vi "Process_DAQ.vi"(8 "error in (no error)":errorcluster, 9 "start process sync notifier":refnum<notifier>, 10 "TopLevel":refnum<class "TopLevel.lvclass">, 11 "DAQ":refnum<class "DAQ.lvclass">) -> (0 "error out":errorcluster)   [LabVIEW 2022 SP3, in "DAQ.lvclass"]
doc: "Developed by Kevin Thompson\nkevin@thompsonengineering.net\n\nCopyright 2015\nThompson Engineering, LLC"
uses:
  DAQ.lvclass
  TopLevel/TopLevel.lvclass
  Process_DAQ SM AppData--cluster.ctl
  DataTypes/TD DAQ Settings--cluster.ctl
  DataTypes/TD DI Instrument Settings--cluster.ctl
  DataTypes/TD AI Instrument Settings--cluster.ctl
  DataTypes/TD AI InstSettings--cluster.ctl
  ProcessSupport/TD SimAI Ranges--cluster.ctl
  <vilib>/TELLC/Dynamic CVT API/TD Dynamic CVT DVR--ref.ctl
  DAQ.lvclass/DAQ.ctl
  ProcessSupport/TD DAQ Output Cmd EventData--cluster.ctl
  ProcessSupport/TD DaqOutCmd--enum.ctl
  DataTypes/TD DAQ Output EventSenderMode-enum.ctl
  DataTypes/TD DO Channel--cluster.ctl
  DataTypes/TD AO Channel--cluster.ctl
  DataTypes/TD DataValueConversion--cluster.ctl
  DataTypes/AsyncCmd_DAQ--enum.ctl
  Accessors/Get AI TaskNames.vi
  Accessors/Get DI TaskNames.vi
  Accessors/Get DAQ Settings.vi
  <vilib>/DAQmx/read.llb/DAQmx Read (Digital Bool 1Line 1Point).vi
  Accessors/Get IO Nodes.vi
  ProcessSupport/Get AI DAQ SMQ - array.vi
  ProcessSupport/Get DI DAQ SMQ - array.vi
  ProcessSupport/Get AI DAQ SMQ - single.vi
  <vilib>/DAQmx/miscellaneous.llb/DAQmx Fill In Error Info.vi
  DAQ_Common/Lib/ErrorHandler/ErrorHandler.lvclass
panel:
  in  "injected error cluster":errorcluster
  in  "inject error":bool
  out "time per buffer":dbl
  in  "Stop Process":bool
  # "Simulated error injection\nfor testing and debug"
  # "Makes sure to set this value from the process caller. Using the Start asyncronous call function."
  # "This is for debugging. Process should stop from user event."
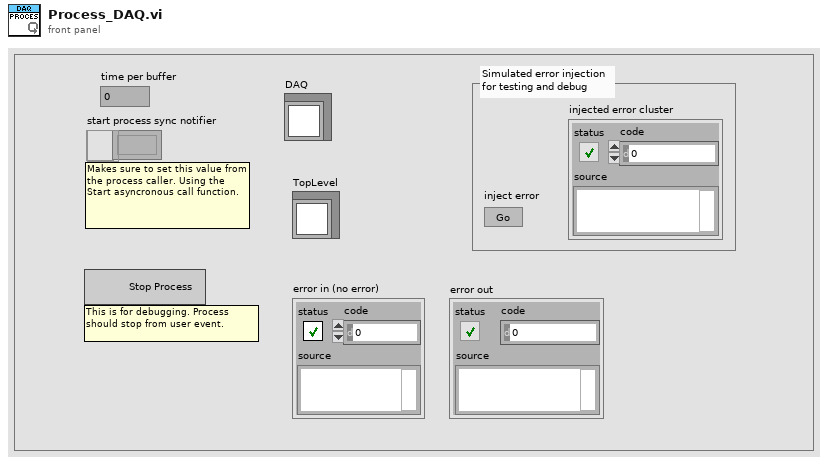
[diagram p1: front panel]
types:
  T1 = typedef "DAQ.lvclass/Process_DAQ SM AppData--cluster.ctl" = cluster{"Core":cluster{"Current VI Ref":refnum<vi>, "process sync notifier":refnum<notifier>}, "AsyncSMQ":refnum<queue>, "DAQ Settings":T2, "SimDaqLoopIntv":i32, "ThreadSyncRndzv":T7, "DAQ Node Dict DVR":T8, "DAQ Data Dict DVR":T8, "vData":variant, "quitting":bool, "Self Reference":refnum<class "DAQ.lvclass">, "AI Thread SMQs":variant, "AI TaskNames*":string[], "AI DAQ SMQ []":refnum<queue>[], "DI Thread SMQs":variant, "DI TaskNames*":string[], "DI DAQ SMQ []":refnum<queue>[]}
  T2 = typedef "DAQ.lvclass/TD DAQ Settings--cluster.ctl" = cluster{"Simulate DAQ":bool, "DI Settings":T3[], "AI Settings":T4[], "Relay IONames":string[], "AO IONames":string[], "AO NChan SingleTask":bool}
  T3 = typedef "DAQ.lvclass/TD DI Instrument Settings--cluster.ctl" = cluster{"Disable":bool, "DI TaskName":string, "DI RefreshIntv":i32}
  T4 = typedef "DAQ.lvclass/TD AI Instrument Settings--cluster.ctl" = cluster{"Disable":bool, "AI TaskName":string, "AI InstSettings":T5, "SimAI Ranges":T6}
  T5 = typedef "DAQ.lvclass/TD AI InstSettings--cluster.ctl" = cluster{"DaqRate":dbl, "NumSamples":i32}
  T6 = typedef "DAQ.lvclass/TD SimAI Ranges--cluster.ctl" = cluster{"lo":dbl, "hi":dbl}
  T7 = typedef "Rendezvous RefNum" = refnum<k1>
  T8 = typedef "TD Dynamic CVT DVR--ref.ctl" = refnum<data-value>
  T9 = typedef "DAQ.lvclass/TD DO Channel--cluster.ctl" = cluster{"DevName":string, "IOName":string, "IOPath":string, "SchemName":string, "logic":enum16{"Lo", "Hi"}, "DAQmx Task":refnum<k21>}
  T10 = typedef "DAQ.lvclass/TD DAQ Output Cmd EventData--cluster.ctl" = cluster{"TimeStamp":dbl, "DaqOutCmd":T11, "IOName":string, "BoolState":bool, "AnalogVal":dbl, "WaitTime (ms)":u32, "mode":T12, "vData":variant}
  T11 = typedef "DAQ.lvclass/TD DaqOutCmd--enum.ctl" = enum16{"Set DO", "Set AO", "Toggle DO", "Invert DO"}
  T12 = typedef "DAQ.lvclass/TD DAQ Output EventSenderMode-enum.ctl" = enum16{"manual", "automation"}
  T13 = typedef "DAQ.lvclass/TD AO Channel--cluster.ctl" = cluster{"DevName":string, "IOName":string, "IOPath":string, "SchemName":string, "Vmin":dbl, "Vmax":dbl, "Conversion":T14, "DAQmx Task":refnum<k21>}
  T14 = typedef "DAQ.lvclass/TD DataValueConversion--cluster.ctl" = cluster{"MaxSignal":dbl, "MinSignal":dbl, "MaxEngUnit":dbl, "MinEngUnit":dbl, "ScaleOffset":dbl, "negate":bool}
  T15 = typedef "DAQ.lvclass/AsyncCmd_DAQ--enum.ctl" = enum16{"StartDAQ", "StopDAQ", "CfgDAQ"}
  T16 = typedef "DAQ.lvclass/TD IO Node Definition--cluster.ctl" = cluster{"DI Config":T17, "DO Config":T20, "AI Config":T21, "AO Config":T26}
  T17 = typedef "DAQ.lvclass/TD DI Config--cluster.ctl" = cluster{"DI Tasks":T18[]}
  T18 = typedef "DAQ.lvclass/TD DI Task--cluster.ctl" = cluster{"DI TaskName":string, "DI Channels":T19[]}
  T19 = typedef "DAQ.lvclass/TD DI Channel--cluster.ctl" = cluster{"DevName":string, "IOName":string, "IOPath":string, "SchemName":string, "logic":enum16{"Lo", "Hi"}, "Index":i32}
  T20 = typedef "DAQ.lvclass/TD DO Config--cluster.ctl" = cluster{"DO Channels":T9[]}
  T21 = typedef "DAQ.lvclass/TD AI Config--cluster.ctl" = cluster{"AI Tasks":T22[]}
  T22 = typedef "DAQ.lvclass/TD AI Task--cluster.ctl" = cluster{"AI TaskName":string, "AI Channels":T23[]}
  T23 = typedef "DAQ.lvclass/TD AI Channel--cluster.ctl" = cluster{"DevName":string, "IOName":string, "IOPath":string, "SchemName":string, "MinValue":dbl, "MaxValue":dbl, "Terminal Configuration":i32, "Index":i32, "Conversion":T14, "AIType":T24, "Force Bridge":T25}
  T24 = typedef "DAQ.lvclass/TD AI DAQ Type--enum.ctl" = enum16{"Voltage", "Current", "Strain Gage", "Force Bridge"}
  T25 = typedef "DAQ.lvclass/TD AI Force Bridge--cluster.ctl" = cluster{"bridge information":cluster{"bridge configuration":i32, "voltage excitation source":i32, "voltage excitation value":dbl, "nominal bridge resistance":dbl}, "scaling information":cluster{"first electrical value":dbl, "second electrical value":dbl, "electrical units":i32, "first physical value":dbl, "second physical value":dbl, "physical units":i32}}
  T26 = typedef "DAQ.lvclass/TD AO Config--cluster.ctl" = cluster{"AO Channels":T13[]}
  T27 = typedef "TopLevel.lvclass/UserEvents.ctl" = cluster{"API Incoming Event":refnum<user-event>, "API Executed Event":refnum<user-event>, "API Return Event":refnum<user-event>, "Exit Event":refnum<user-event>, "StatusChanged":refnum<user-event>, "DLP GUI Config Changed":refnum<user-event>, "AppEvent":refnum<user-event>, "Login Event":refnum<user-event>, "HeadPrimeStatusEvent":refnum<user-event>}
  T28 = typedef "DAQ.lvclass/TD PublicEvents--cluster.ctl" = cluster{"DaqOutputCmd Ev":refnum<user-event>, "stop process":refnum<user-event>, "DAQ.AsyncCmd Event":refnum<user-event>, "DAQStateChanged Event":refnum<user-event>, "DAQ.AsyncMsg Event":refnum<user-event>, "DAQ_DO_StatusEvent":refnum<user-event>, "DIStateChangeEv":refnum<user-event>, "UI StateChanged":refnum<user-event>, "PurgeTimerEvent":refnum<user-event>}
  T29 = cluster{"AI InstSettings":T5, "AI TaskName":string}
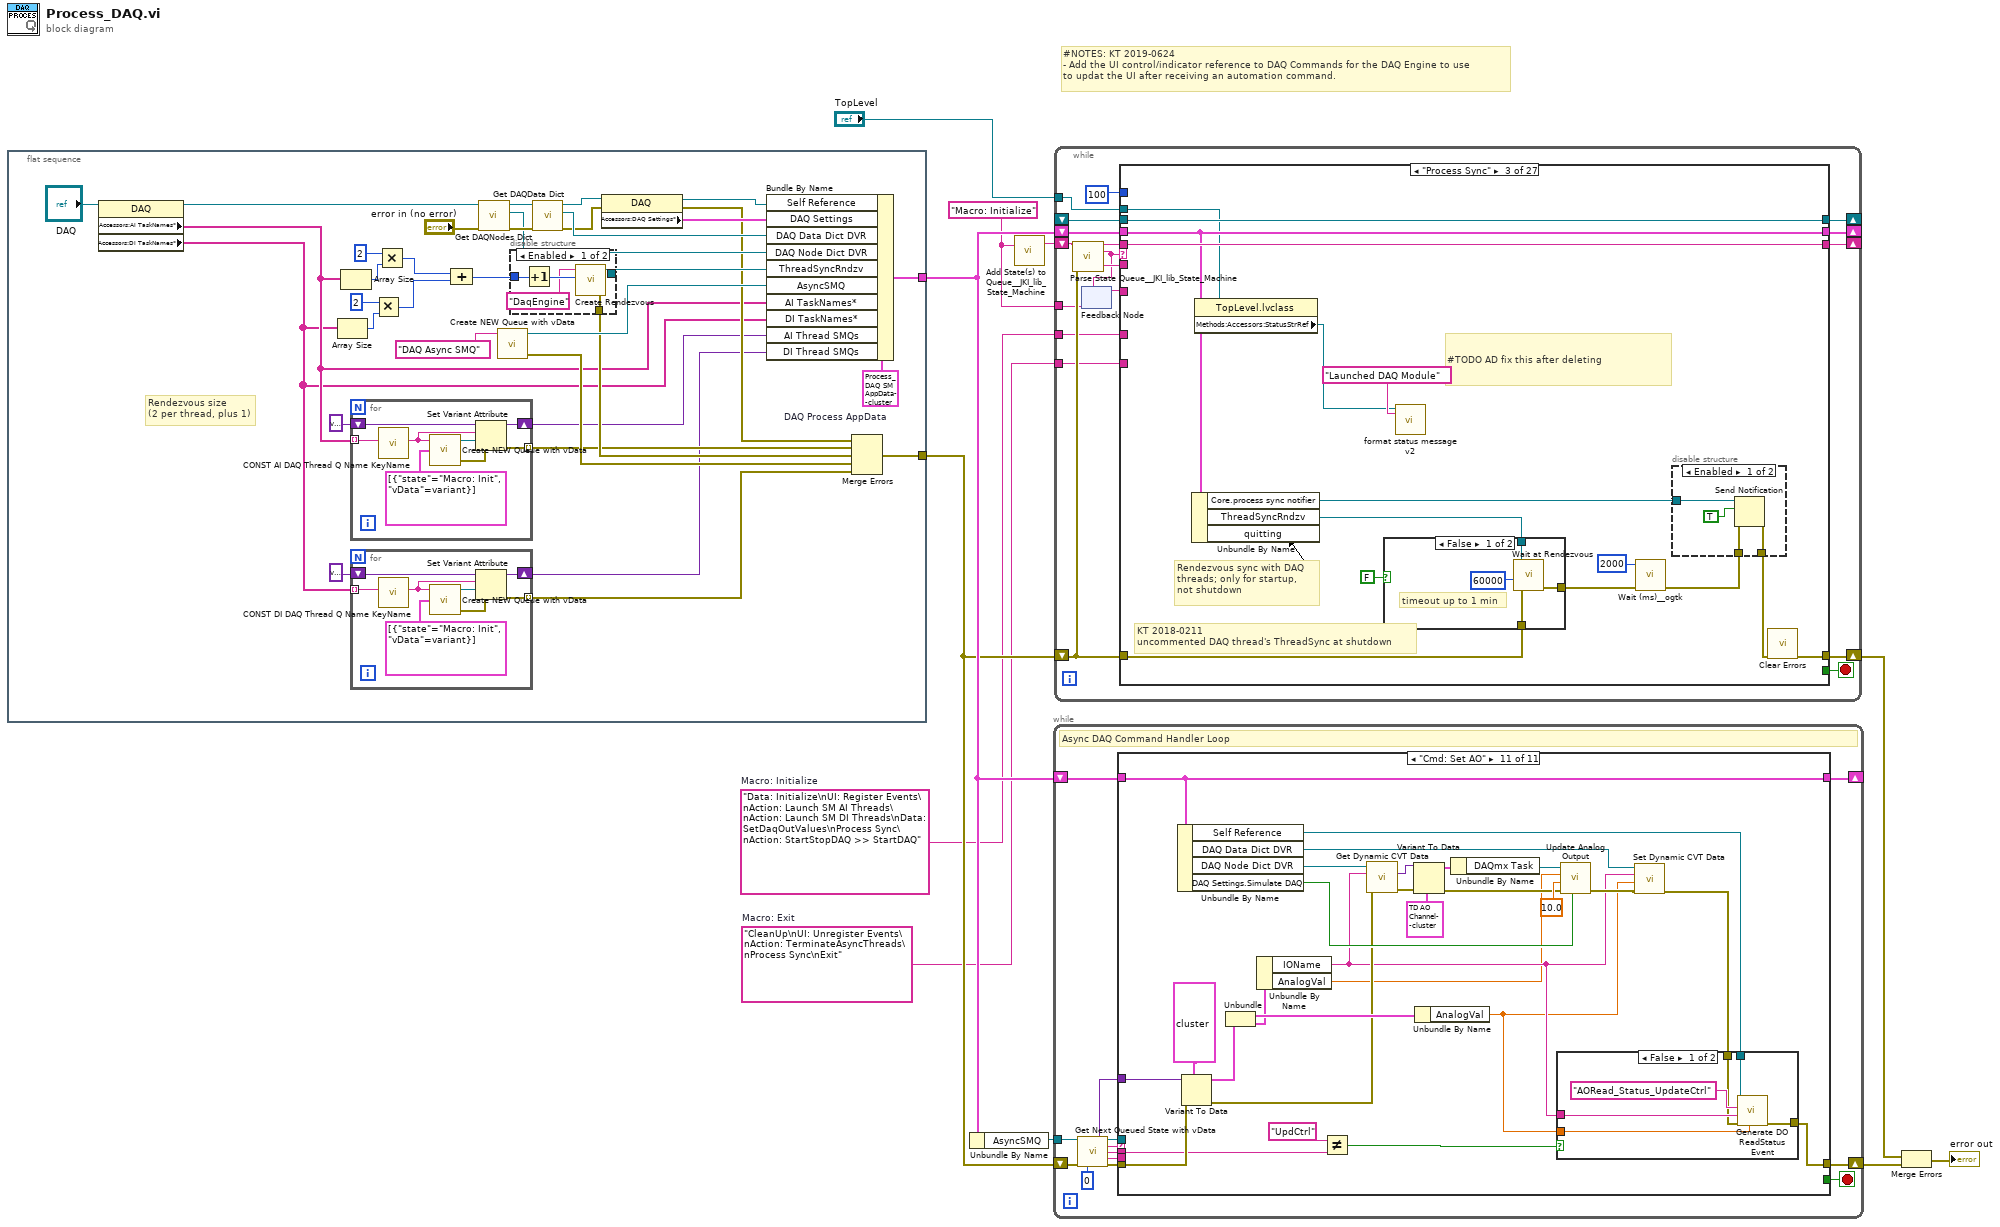
[diagram p0: block diagram]
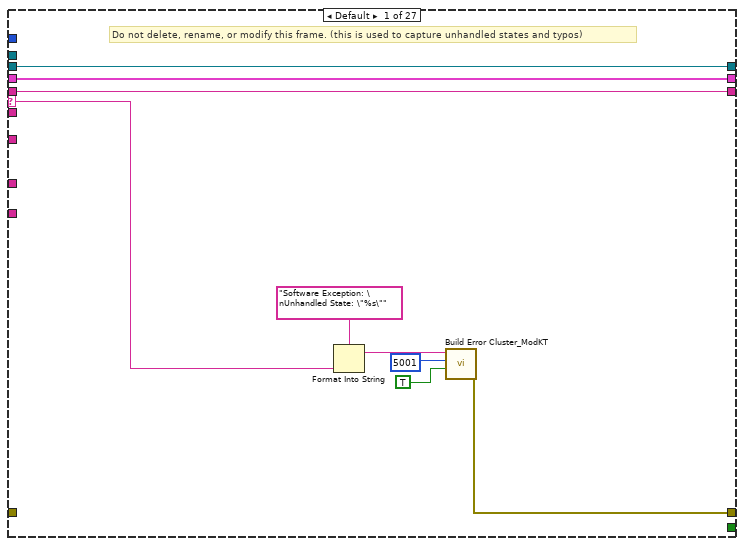
[diagram p2: hidden frame]
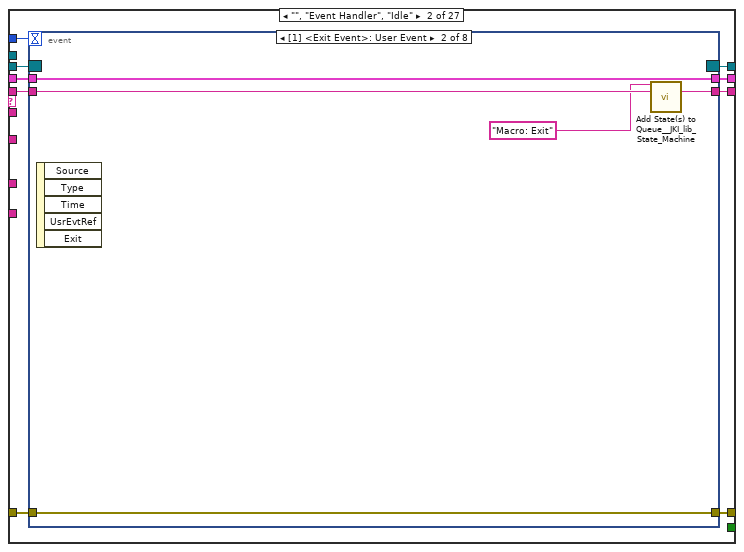
[diagram p3: hidden frame]
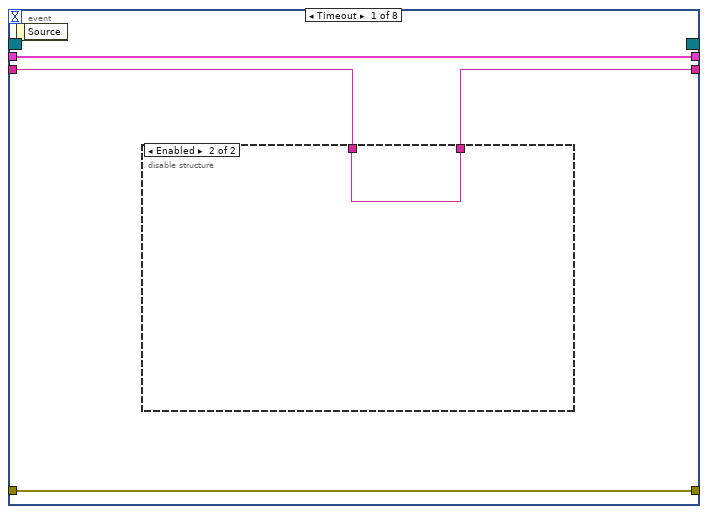
[diagram p4: hidden frame]
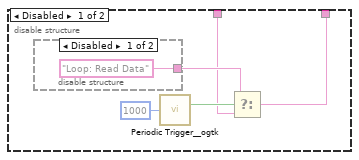
[diagram p5: hidden frame]
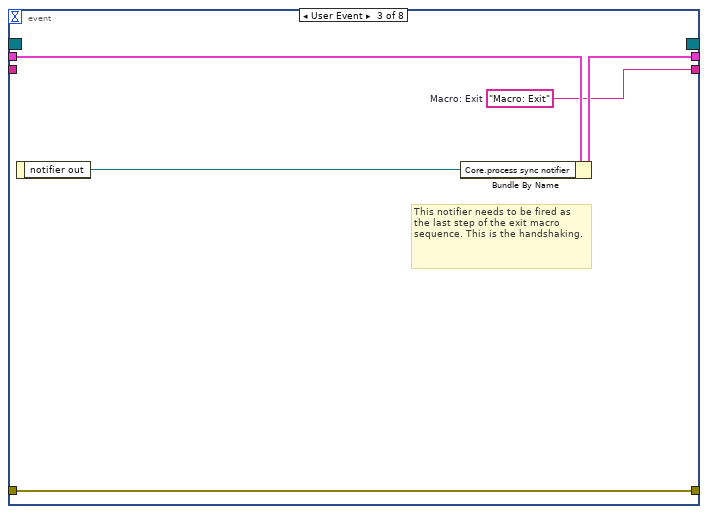
[diagram p7: hidden frame]
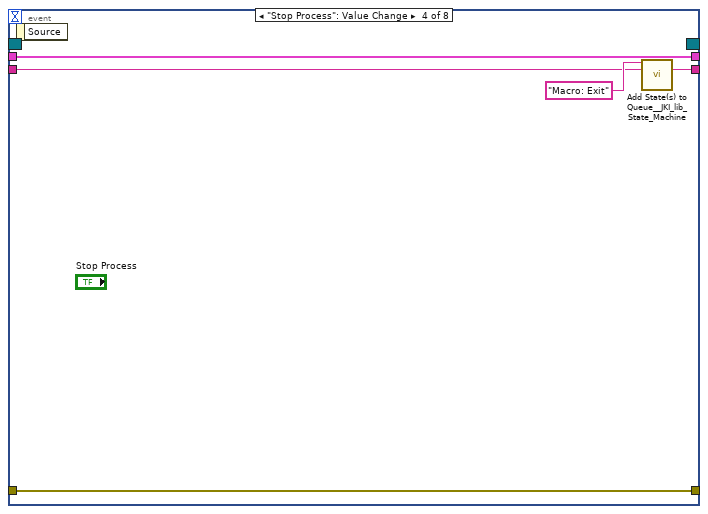
[diagram p8: hidden frame]
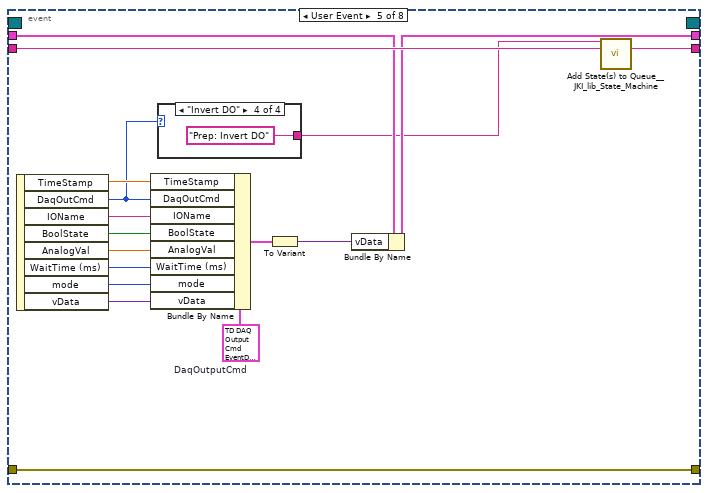
[diagram p9: hidden frame]
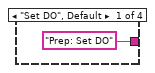
[diagram p10: hidden frame]
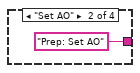
[diagram p11: hidden frame]
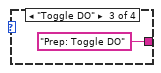
[diagram p12: hidden frame]
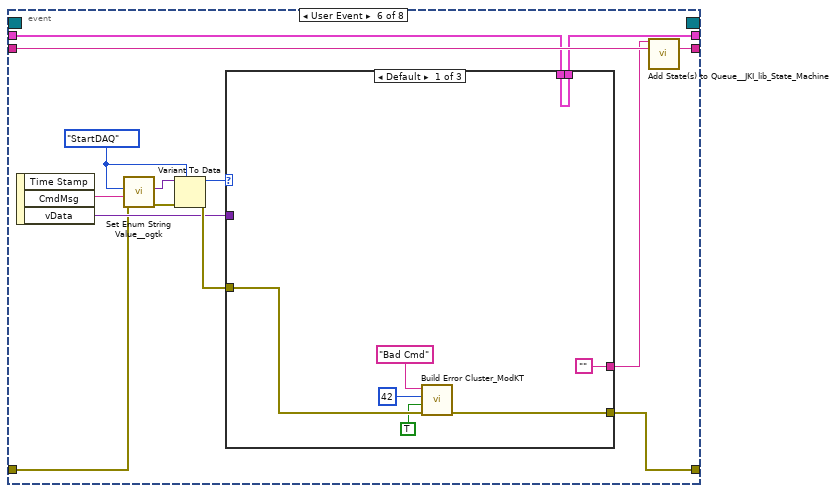
[diagram p13: hidden frame]
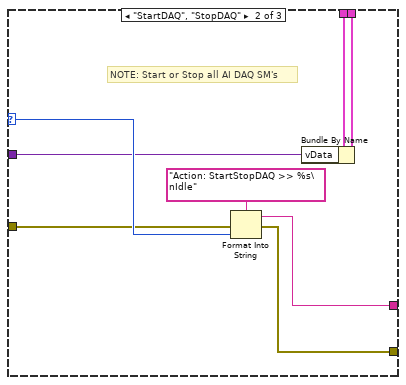
[diagram p14: hidden frame]
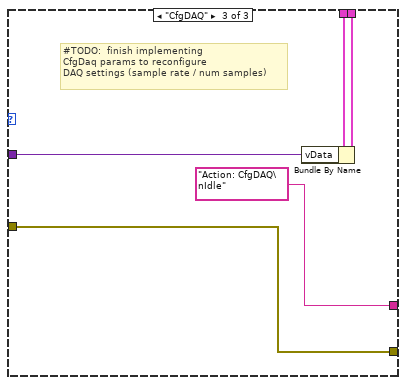
[diagram p15: hidden frame]
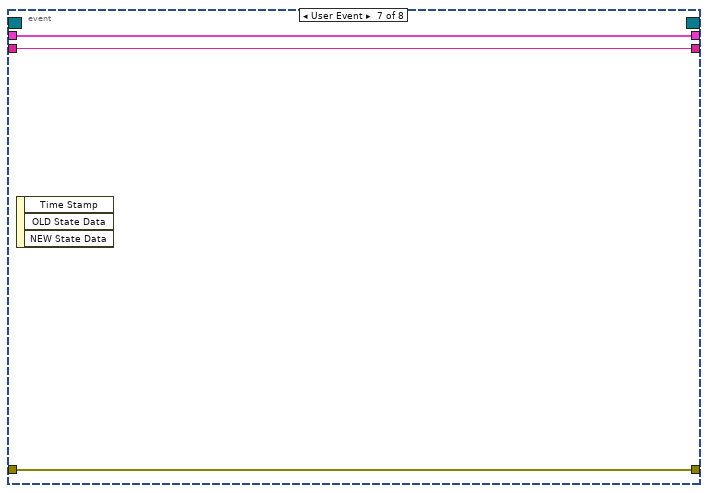
[diagram p16: hidden frame]
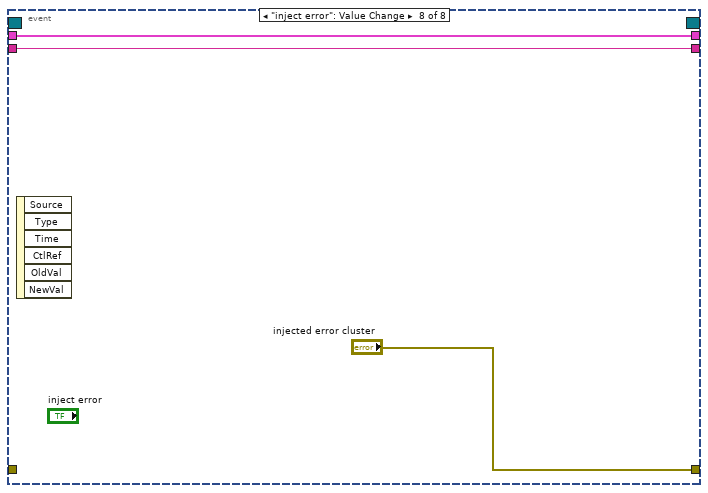
[diagram p17: hidden frame]
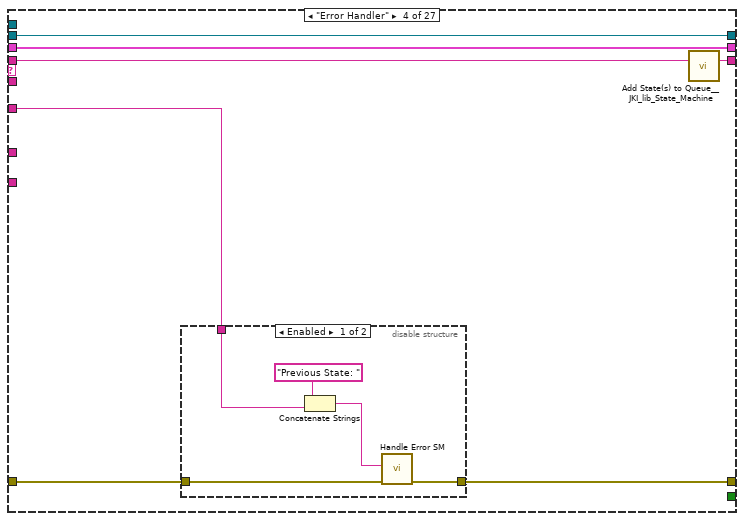
[diagram p20: hidden frame]
diagram:
  w4 = "Data: Initialize\nUI: Register Events\nAction: Launch SM AI Threads\nAction: Launch SM DI Threads\nData: SetDaqOutValues\nProcess Sync\nAction: StartStopDAQ >> StartDAQ"  # Macro: Initialize
  w3 = "CleanUp\nUI: Unregister Events\nAction: TerminateAsyncThreads\nProcess Sync\nExit"  # Macro: Exit
  w2 = "Macro: Initialize"
  # "#NOTES: KT 2019-0624\n- Add the UI control/indicator reference to DAQ Commands for the DAQ Engine to use\nto updat the UI after receiving an automation command."
  n1 = flat-sequence {
    tunnel: [w45] -> w9
    tunnel: [w35] -> w8
    frame #0 {
      w46 = T1 {"Core"={"Current VI Ref"=refnum, "process sync notifier"=refnum}, "AsyncSMQ"=refnum, "DAQ Settings"={"Simulate DAQ"=FALSE, "DI Settings"=[], "AI Settings"=[], "Relay IONames"=[], "AO IONames"=[], "AO NChan SingleTask"=FALSE}, "SimDaqLoopIntv"=0, "ThreadSyncRndzv"=refnum, "DAQ Node Dict DVR"=refnum, "DAQ Data Dict DVR"=refnum, "vData"=variant, "quitting"=FALSE, "Self Reference"=refnum, "AI Thread SMQs"=variant, "AI TaskNames*"=[], "AI DAQ SMQ []"=[], "DI Thread SMQs"=variant, "DI TaskNames*"=[], "DI DAQ SMQ []"=[]}  # DAQ Process AppData
      # "Rendezvous size\n(2 per thread, plus 1)"
      n2 = property class="DAQ"(reference="DAQ") -> (reference out=w26:refnum<class "DAQ.lvclass">, "Accessors:AI TaskNames*"=w23:string[], "Accessors:DI TaskNames*"=w13:string[])  [unwired: 1 in, 1 out]
      n3 = Array Size(array=w13) -> (size(s)=w18:i32)
      n4 = Array Size(array=w23) -> (size(s)=w22:i32)
      n5 = for {
        tunnel: [w65] -> w32 mode=indexing
        shift-right: [w64] -> w24
        shift-left: variant -> [w66]
        tunnel: w23 -> [w61] mode=indexing
        n6 = call "CONST AI DAQ Thread Q Name KeyName.vi"("AI TaskName"=w61) -> ("AI SMQ (KeyName)"=w63:string)  [unwired: 10 in]
        n7 = call <vilib>:"Create NEW Queue with vData.vi"("Initial States"=cluster{"state":string, "vData":variant}[] [{"state"="Macro: Init", "vData"=variant}], "Name (SMQ)"=w63) -> ("error out"=w60:errorcluster, "queue out"=w67:refnum<queue>)  [unwired: 2 in]
        n8 = Set Variant Attribute(Variant=w66, name=w63, value=w67, error in=w60) -> (Variant out=w64:variant, error out=w65:errorcluster)  [unwired: 1 out]
      }
      n9 = for {
        tunnel: [w57] -> w14 mode=indexing
        shift-right: [w56] -> w12
        shift-left: variant -> [w58]
        tunnel: w13 -> [w53] mode=indexing
        n10 = call "CONST DI DAQ Thread Q Name KeyName.vi"("DI TaskName"=w53) -> ("DI SMQ (KeyName)"=w55:string)  [unwired: 10 in]
        n11 = call <vilib>:"Create NEW Queue with vData.vi"("Initial States"=cluster{"state":string, "vData":variant}[] [{"state"="Macro: Init", "vData"=variant}], "Name (SMQ)"=w55) -> ("error out"=w52:errorcluster, "queue out"=w59:refnum<queue>)  [unwired: 2 in]
        n12 = Set Variant Attribute(Variant=w58, name=w55, value=w59, error in=w52) -> (Variant out=w56:variant, error out=w57:errorcluster)  [unwired: 1 out]
      }
      n13 = Multiply(x=2, y=w18) -> (x*y=w16:i32)
      n14 = Multiply(x=2, y=w22) -> (x*y=w20:i32)
      n15 = Compound Arithmetic op=ADD(w20, w16) -> (w17:i32)
      n16 = call "Get DAQNodes Dict.vi"("error in (no error)"="error in (no error)", "DAQ"=w26) -> ("error out"=w39:errorcluster, "DAQ Node Dict DVR"=w38:T8, "DAQ"=w41:refnum<class "DAQ.lvclass">)  [unwired: 7 in]
      n17 = call <vilib>:"Create NEW Queue with vData.vi"("Name (SMQ)"="DAQ Async SMQ") -> ("error out"=w43:errorcluster, "queue out"=w42:refnum<queue>)  [unwired: 3 in]
      n18 = disable-structure shown="Enabled" {
        disable-tunnel: [w51 _] -> w37
        disable-tunnel: [w50 _] -> w36
        disable-tunnel: w17 -> [w47 _]
        frame Enabled {
          n19 = Increment(x=w47) -> (x+1=w49:i32)
          n20 = call <vilib>:"Create Rendezvous.vi"("size (2)"=w49, "name (unnamed)"="DaqEngine" ("ProcVI ID")) -> ("error out"=w50:errorcluster, "rendezvous"=w51:T7)  [unwired: 3 in, 1 out]
        }
        frame Disabled {
        }
      }
      n21 = call "Get DAQData Dict.vi"("error in (no error)"=w39, "DAQ"=w41) -> ("error out"=w28:errorcluster, "DAQ Data Dict DVR"=w40:T8, "DAQ"=w31:refnum<class "DAQ.lvclass">)  [unwired: 7 in]
      n22 = property class="DAQ"(reference=w31, error in=w28) -> (reference out=w29:refnum<class "DAQ.lvclass">, error out=w25:errorcluster, "Accessors:DAQ Settings*"=w30:T2)
      n23 = Bundle By Name(cluster=w46, "Self Reference"=w29, "DAQ Settings"=w30, "DAQ Data Dict DVR"=w40, "DAQ Node Dict DVR"=w38, "ThreadSyncRndzv"=w37, "AsyncSMQ"=w42, "AI TaskNames*"=w23, "DI TaskNames*"=w13, "AI Thread SMQs"=w24, "DI Thread SMQs"=w12) -> (w45:T1)
      n24 = Merge Errors(w25, w32, w36, w43, w14) -> (w35:errorcluster)
    }
  }
  n25 = Unbundle By Name(w9) -> ("AsyncSMQ"=w10:refnum<queue>)
  n26 = call <vilib>:"Add State(s) to Queue__JKI_lib_State_Machine.vi"("State(s) in (\"\")"=w2) -> ("States Out"=w11:string)  [unwired: 14 in]
  n27 = while {
    shift-right: [w69] -> _
    shift-left: w9 -> [w70]
    tunnel: w10 -> [w80]
    shift-right: [w72] -> w7
    shift-left: w8 -> [w74]
    stop <- w71 stop-if-true
    # "Async DAQ Command Handler Loop"
    n28 = call <vilib>:"Get Next Queued State with vData.vi"("queue in"=w80, "error in (no error)"=w74, "timeout (100)"=0) -> ("vData out"=w75:variant, "queue out"=w78:refnum<queue>, "Next State"=w79:string, "queued msg"=w77:string, "Prev State"=w76:string, "error out"=w73:errorcluster)  [unwired: 6 in, 1 out]
    n29 = case shown="\"Cmd: Set AO\"" w79 {
      tunnel: w73 -> [_ w90 w100 _ w108 w115 w118 w138 w182 w228 w272]
      tunnel: w78 -> [_ _ _ w104 w109 _ _ _ _ _ _]
      tunnel: w77 -> [_ _ _ _ _ _ _ w134 w178 w224 w252]
      selector: w79 -> [w81 _ _ _ _ _ _ _ _ _ _]
      tunnel: w76 -> [_ w89 _ _ _ _ _ _ _ _ _]
      tunnel: w75 -> [_ _ _ _ _ _ _ w139 w183 w229 w271]
      tunnel: [w82 w88 w100 w106 w108 w114 w118 w122 w171 w215 w247] -> w72
      tunnel: [_ _ _ _ TRUE _ _ _ _ _ _] -> w71
      tunnel: w70 -> [w87 w91 w99 w107 w111 w116 w117 w137 w181 w227 w255]
      tunnel: [w87 w91 w99 w107 w111 w116 w117 w137 w181 w227 w255] -> w69
      frame Default {
        n30 = Format Into String(format string="Software Exception: \nUnhandled State: \"%s\"", w81) -> (resulting string=w84:string)  [unwired: 2 in, 1 out]
        n31 = call <vilib>:"Build Error Cluster_ModKT .vi"("Prepend String (\"\")"=w84, "code"=5001, "error? (F)"=TRUE ("error?")) -> ("error out"=w82:errorcluster)  [unwired: 4 in, 1 out]
      }
      frame "Error Handler" {
        n32 = disable-structure shown="Enabled" {
          disable-tunnel: w90 -> [w94 w98]
          disable-tunnel: w89 -> [w93 _]
          disable-tunnel: [w92 errorcluster {"status"=FALSE, "code"=0, "source"=""} ("error constant")] -> w88
          frame Enabled {
            n33 = Concatenate Strings("Previous State: ", w93) -> (w96:string)
            n34 = call "Handle Error SM.vi"("error in (no error)"=w94, "CustomMessage"=w96) -> ("error out"=w92:errorcluster)  [unwired: 7 in, 2 out]
          }
          frame Disabled {
            n35 = call <vilib>:"General Error Handler.vi"("error in (no error)"=w98) -> ()  [unwired: 10 in, 5 out]
          }
        }
      }
      frame "Initialize" {
      }
      frame "CleanUp", "Macro: Exit" {
        # "Do any necessary async loop clean up here before quitting"
        n36 = Flush Queue(queue=w104, error in (no error)=errorcluster {"status"=FALSE, "code"=0, "source"=""}) -> (queue out=w105:refnum<queue>, error out=w103:errorcluster)  [unwired: 1 out]
        n37 = call <vilib>:"Add State to Queue with vData.vi"("queue in"=w105, "state in"="Exit", "error in"=w103) -> ("error out"=w106:errorcluster)  [unwired: 9 in, 3 out]
      }
      frame "Exit", "Quit" {
        n38 = Release Queue(queue=w109, force destroy? (F)=TRUE) -> ()  [unwired: 1 in, 3 out]
      }
      frame "", "Idle" {
        n39 = call <userlib>:"Wait (ms)__ogtk.vi"("error in (no error)"=w115, "milliseconds to wait"=u32 100) -> ("error out"=w114:errorcluster)  [unwired: 8 in, 1 out]
      }
      frame "------ Cmd ------" {
      }
      frame "Cmd: Set DO" {
        # "\"Fire Update UI Control Value Change Event.vi\""
        # "Bypass updating UI control if not \nautomation mode."
        n40 = Unbundle By Name(w137) -> ("Self Reference"=w124:refnum<class "DAQ.lvclass">, "DAQ Data Dict DVR"=w146:T8, "DAQ Node Dict DVR"=w140:T8, "DAQ Settings.Simulate DAQ"=w148:bool)
        n41 = Variant To Data(error in=w138, type=cluster{"CmdOrig":T10, "CmdCnvrt":T10} {"CmdOrig"={"TimeStamp"=0.0, "DaqOutCmd"=enum."Set DO", "IOName"="", "BoolState"=FALSE, "AnalogVal"=0.0, "WaitTime (ms)"=0, "mode"=enum."manual", "vData"=variant}, "CmdCnvrt"={"TimeStamp"=0.0, "DaqOutCmd"=enum."Set DO", "IOName"="", "BoolState"=FALSE, "AnalogVal"=0.0, "WaitTime (ms)"=0, "mode"=enum."manual", "vData"=variant}}, Variant=w139) -> (data=w151:cluster{"CmdOrig":T10, "CmdCnvrt":T10}, error out=w147:errorcluster)
        n42 = Unbundle(w151) -> ("CmdOrig"=w150:T10, "CmdCnvrt"=w149:T10)
        n43 = Unbundle By Name(w149) -> ("IOName"=w121:string, "BoolState"=w130:bool)
        n44 = call <vilib>:"Get Dynamic CVT Data.vi"("error in (no error)"=w147, "DataName"=w121, "dCVT DVR"=w140) -> ("error out"=w141:errorcluster, "value"=w142:variant)  [unwired: 5 in, 2 out]
        n45 = Unbundle By Name(w150) -> ("BoolState"=w133:bool, "WaitTime (ms)"=w131:u32)
        n46 = Variant To Data(error in=w141, type=T9 {"DevName"="", "IOName"="", "IOPath"="", "SchemName"="", "logic"=enum."Lo", "DAQmx Task"=""} ("DO"), Variant=w142) -> (data=w143:T9, error out=w129:errorcluster)
        n47 = Unbundle By Name(w143) -> ("DAQmx Task"=w144:refnum<k21>)
        n48 = Not Equal?(x="UpdCtrl", y=w134) -> (x != y?=w120:bool)
        n49 = call "Actuate Digital Line.vi"("Simulate"=w148, "error in"=w129, "timeout"=10.0, "state"=w130, "DO-Line Ref"=w144) -> ("error out"=w127:errorcluster, "DO-Line Ref out"=w128:refnum<k21>)  [unwired: 5 in]
        n50 = case shown="False" w120 {
          tunnel: ["DORead_Status_UpdateCtrl" ("CmdMsg") "DORead_Status" ("CmdMsg")] -> w119
          frame False {
          }
          frame True {
          }
        }
        n51 = disable-structure shown="Enabled" {
          disable-tunnel: w121 -> [_ _]
          disable-tunnel: w133 -> [_ _]
          disable-tunnel: w127 -> [w159 w160]
          disable-tunnel: [w156 w160] -> w132
          disable-tunnel: w128 -> [w158 _]
          disable-tunnel: [w155 _] -> w126
          frame Enabled {
            n52 = call-poly <vilib>:"DAQmx Read.vi"("task/channels in"=w158, "timeout"=10.0, "error in"=w159) -> ("data"=w155:bool, "error out"=w156:errorcluster)  [unwired: 10 in, 1 out]
          }
          frame Disabled {
          }
        }
        n53 = call <userlib>:"Wait (ms)__ogtk.vi"("error in (no error)"=w132, "milliseconds to wait"=w131) -> ("error out"=w125:errorcluster)  [unwired: 8 in, 1 out]
        n54 = call <vilib>:"Set Dynamic CVT Data.vi"("error in (no error)"=w125, "value"=w126, "DataName"=w121, "dCVT DVR"=w146) -> ("error out"=w123:errorcluster)  [unwired: 5 in, 2 out]
        n55 = call "Generate DO ReadStatus Event.vi"("error in (no error)"=w123, "DO IOName"=w121, "CmdMsg"=w119, "DAQ"=w124) -> ("error out"=w122:errorcluster)  [unwired: 6 in, 1 out]
      }
      frame "Cmd: Toggle DO" {
        # "#NOTE: consider using the event data's vData element for toggle delay intervals"
        # "\"Fire Update UI Control Value Change Event.vi\""
        # "Bypass updating UI control if not \nautomation mode."
        n56 = Unbundle By Name(w181) -> ("DAQ Data Dict DVR"=w188:T8, "DAQ Node Dict DVR"=w184:T8, "DAQ Settings.Simulate DAQ"=w166:bool)
        n57 = Variant To Data(error in=w182, type=cluster{"CmdOrig":T10, "CmdCnvrt":T10} {"CmdOrig"={"TimeStamp"=0.0, "DaqOutCmd"=enum."Set DO", "IOName"="", "BoolState"=FALSE, "AnalogVal"=0.0, "WaitTime (ms)"=0, "mode"=enum."manual", "vData"=variant}, "CmdCnvrt"={"TimeStamp"=0.0, "DaqOutCmd"=enum."Set DO", "IOName"="", "BoolState"=FALSE, "AnalogVal"=0.0, "WaitTime (ms)"=0, "mode"=enum."manual", "vData"=variant}}, Variant=w183) -> (data=w192:cluster{"CmdOrig":T10, "CmdCnvrt":T10}, error out=w189:errorcluster)
        n58 = Unbundle(w192) -> ("CmdOrig"=w191:T10, "CmdCnvrt"=w190:T10)
        n59 = Unbundle By Name(w190) -> ("IOName"=w172:string, "BoolState"=w168:bool)
        n60 = Not Equal?(x="UpdCtrl", y=w178) -> (x != y?=w176:bool)
        n61 = call <vilib>:"Get Dynamic CVT Data.vi"("error in (no error)"=w189, "DataName"=w172, "dCVT DVR"=w184) -> ("error out"=w185:errorcluster, "value"=w186:variant)  [unwired: 5 in, 2 out]
        n62 = Unbundle By Name(w191) -> ("BoolState"=w177:bool, "WaitTime (ms)"=w173:u32, "vData"=w165:variant)
        n63 = Variant To Data(error in=w185, type=T9 {"DevName"="", "IOName"="", "IOPath"="", "SchemName"="", "logic"=enum."Lo", "DAQmx Task"=""} ("DO"), Variant=w186) -> (data=w187:T9, error out=w162:errorcluster)
        n64 = Unbundle By Name(w187) -> ("DAQmx Task"=w170:refnum<k21>)
        n65 = disable-structure shown="Disabled" {
          disable-tunnel: w162 -> [w195 w197]
          disable-tunnel: [w194 w197] -> w161
          frame Disabled {
            n66 = call <userlib>:"Wait (ms)__ogtk.vi"("error in (no error)"=w195, "milliseconds to wait"=u32 250) -> ("error out"=w194:errorcluster)  [unwired: 8 in, 1 out]
          }
          frame Enabled {
          }
        }
        n67 = Variant To Data(type=u32 250 ("ToggleWaitIntv (250ms)"), Variant=w165) -> (data=w163:u32)  [unwired: 1 in, 1 out]
        n68 = call "Toggle Relay.vi"("Simulate"=w166, "timeout"=10.0, "error in"=w161, "InitialState (T)"=w168, "ToggleWaitIntv (250ms)"=w163, "DO-Line Ref"=w170) -> ("error out"=w169:errorcluster)  [unwired: 4 in, 1 out]
        n69 = call <vilib>:"Set Dynamic CVT Data.vi"("error in (no error)"=w169, "value"=w177, "DataName"=w172, "dCVT DVR"=w188) -> ("error out"=w175:errorcluster)  [unwired: 5 in, 2 out]
        n70 = disable-structure shown="Enabled" {
          disable-tunnel: w172 -> [w201 _]
          disable-tunnel: w177 -> [w200 _]
          disable-tunnel: w176 -> [w199 _]
          disable-tunnel: w175 -> [w198 w202]
          disable-tunnel: [w198 w202] -> w174
          frame Disabled {
          }
          frame Enabled {
          }
        }
        n71 = call <userlib>:"Wait (ms)__ogtk.vi"("error in (no error)"=w174, "milliseconds to wait"=w173) -> ("error out"=w171:errorcluster)  [unwired: 8 in, 1 out]
      }
      frame "Cmd: Invert DO" {
        # "#NOTE: consider using the event data's vData element for toggle delay intervals"
        # "\"Fire Update UI Control Value Change Event.vi\""
        # "Bypass updating UI control if not \nautomation mode."
        n72 = Unbundle By Name(w227) -> ("Self Reference"=w217:refnum<class "DAQ.lvclass">, "DAQ Data Dict DVR"=w214:T8, "DAQ Node Dict DVR"=w230:T8, "DAQ Settings.Simulate DAQ"=w207:bool)
        n73 = Variant To Data(error in=w228, type=cluster{"CmdOrig":T10, "CmdCnvrt":T10} {"CmdOrig"={"TimeStamp"=0.0, "DaqOutCmd"=enum."Set DO", "IOName"="", "BoolState"=FALSE, "AnalogVal"=0.0, "WaitTime (ms)"=0, "mode"=enum."manual", "vData"=variant}, "CmdCnvrt"={"TimeStamp"=0.0, "DaqOutCmd"=enum."Set DO", "IOName"="", "BoolState"=FALSE, "AnalogVal"=0.0, "WaitTime (ms)"=0, "mode"=enum."manual", "vData"=variant}}, Variant=w229) -> (data=w237:cluster{"CmdOrig":T10, "CmdCnvrt":T10}, error out=w234:errorcluster)
        n74 = Unbundle(w237) -> ("CmdOrig"=w236:T10, "CmdCnvrt"=w235:T10)
        n75 = Unbundle By Name(w235) -> ("IOName"=w213:string)
        n76 = Not Equal?(x="UpdCtrl", y=w224) -> (x != y?=w205:bool)
        n77 = call <vilib>:"Get Dynamic CVT Data.vi"("error in (no error)"=w234, "DataName"=w213, "dCVT DVR"=w230) -> ("error out"=w231:errorcluster, "value"=w232:variant)  [unwired: 5 in, 2 out]
        n78 = Unbundle By Name(w236) -> ("WaitTime (ms)"=w222:u32, "vData"=w221:variant)  [unwired: 1 out]
        n79 = Variant To Data(error in=w231, type=T9 {"DevName"="", "IOName"="", "IOPath"="", "SchemName"="", "logic"=enum."Lo", "DAQmx Task"=""} ("DO"), Variant=w232) -> (data=w233:T9, error out=w219:errorcluster)
        n80 = Unbundle By Name(w233) -> ("DAQmx Task"=w211:refnum<k21>)
        n81 = disable-structure shown="Disabled" {
          disable-tunnel: w219 -> [w242 w244]
          disable-tunnel: [w241 w244] -> w209
          frame Disabled {
            n82 = call <userlib>:"Wait (ms)__ogtk.vi"("error in (no error)"=w242, "milliseconds to wait"=u32 250) -> ("error out"=w241:errorcluster)  [unwired: 8 in, 1 out]
          }
          frame Enabled {
          }
        }
        n83 = Variant To Data(type=u32 250 ("ToggleWaitIntv (250ms)"), Variant=w221) -> ()  [unwired: 1 in, 2 out]
        n84 = call "Invert Relay.vi"("Simulate"=w207, "timeout"=10.0, "error in"=w209, "DO-Line Ref"=w211) -> ("error out"=w208:errorcluster, "DO-Line Ref out"=w210:refnum<k21>)  [unwired: 6 in]
        n85 = case shown="True" w205 {
          tunnel: ["DORead_Status_UpdateCtrl" ("CmdMsg") "DORead_Status" ("CmdMsg")] -> w203
          frame False {
          }
          frame True {
          }
        }
        n86 = call-poly <vilib>:"DAQmx Read.vi"("task/channels in"=w210, "timeout"=10.0, "error in"=w208) -> ("data"=w212:bool, "error out"=w223:errorcluster)  [unwired: 10 in, 1 out]
        n87 = call <userlib>:"Wait (ms)__ogtk.vi"("error in (no error)"=w223, "milliseconds to wait"=w222) -> ("error out"=w216:errorcluster)  [unwired: 8 in, 1 out]
        n88 = call <vilib>:"Set Dynamic CVT Data.vi"("error in (no error)"=w216, "value"=w212, "DataName"=w213, "dCVT DVR"=w214) -> ("error out"=w218:errorcluster)  [unwired: 5 in, 2 out]
        n89 = call "Generate DO ReadStatus Event.vi"("error in (no error)"=w218, "DO IOName"=w213, "CmdMsg"=w203, "DAQ"=w217) -> ("error out"=w215:errorcluster)  [unwired: 6 in, 1 out]
      }
      frame "Cmd: Set AO" {
        n90 = Unbundle By Name(w255) -> ("Self Reference"=w250:refnum<class "DAQ.lvclass">, "DAQ Data Dict DVR"=w257:T8, "DAQ Node Dict DVR"=w260:T8, "DAQ Settings.Simulate DAQ"=w267:bool)
        n91 = Variant To Data(error in=w272, type=cluster{"CmdOrig":T10, "CmdCnvrt":T10} {"CmdOrig"={"TimeStamp"=0.0, "DaqOutCmd"=enum."Set DO", "IOName"="", "BoolState"=FALSE, "AnalogVal"=0.0, "WaitTime (ms)"=0, "mode"=enum."manual", "vData"=variant}, "CmdCnvrt"={"TimeStamp"=0.0, "DaqOutCmd"=enum."Set DO", "IOName"="", "BoolState"=FALSE, "AnalogVal"=0.0, "WaitTime (ms)"=0, "mode"=enum."manual", "vData"=variant}}, Variant=w271) -> (data=w262:cluster{"CmdOrig":T10, "CmdCnvrt":T10}, error out=w253:errorcluster)
        n92 = Unbundle(w262) -> ("CmdOrig"=w269:T10, "CmdCnvrt"=w268:T10)
        n93 = Unbundle By Name(w268) -> ("IOName"=w249:string, "AnalogVal"=w246:dbl)
        n94 = Not Equal?(x="UpdCtrl", y=w252) -> (x != y?=w251:bool)
        n95 = call <vilib>:"Get Dynamic CVT Data.vi"("error in (no error)"=w253, "DataName"=w249, "dCVT DVR"=w260) -> ("error out"=w258:errorcluster, "value"=w259:variant)  [unwired: 5 in, 2 out]
        n96 = Variant To Data(error in=w258, type=T13 {"DevName"="", "IOName"="", "IOPath"="", "SchemName"="", "Vmin"=0.0, "Vmax"=0.0, "Conversion"={"MaxSignal"=0.0, "MinSignal"=0.0, "MaxEngUnit"=0.0, "MinEngUnit"=0.0, "ScaleOffset"=0.0, "negate"=FALSE}, "DAQmx Task"=""} ("AO"), Variant=w259) -> (data=w263:T13, error out=w265:errorcluster)
        n97 = Unbundle By Name(w269) -> ("AnalogVal"=w245:dbl)
        n98 = Unbundle By Name(w263) -> ("DAQmx Task"=w264:refnum<k21>)
        n99 = call "Update Analog Output.vi"("Simulate"=w267, "error in"=w265, "timeout"=10.0, "AnalogVal in"=w246, "AO Ref"=w264) -> ("error out"=w256:errorcluster)  [unwired: 4 in, 2 out]
        n100 = call <vilib>:"Set Dynamic CVT Data.vi"("error in (no error)"=w256, "value"=w245, "DataName"=w249, "dCVT DVR"=w257) -> ("error out"=w248:errorcluster)  [unwired: 5 in, 2 out]
        n101 = case shown="False" w251 {
          tunnel: w250 -> [w278 _]
          tunnel: w249 -> [w276 _]
          tunnel: w245 -> [w275 _]
          tunnel: w248 -> [w274 w279]
          tunnel: [w273 w279] -> w247
          frame False {
            n102 = call "Generate DO ReadStatus Event.vi"("vData"=w275, "error in (no error)"=w274, "DO IOName"=w276, "CmdMsg"="AORead_Status_UpdateCtrl", "DAQ"=w278) -> ("error out"=w273:errorcluster)  [unwired: 5 in, 1 out]
          }
          frame True {
          }
        }
      }
    }
  }
  n103 = while {
    shift-right: [w291] -> _
    shift-left: w9 -> [w290]
    shift-right: [w294] -> w6
    shift-left: w8 -> [w289]
    shift-right: [w293] -> _
    shift-left: w11 -> [w295]
    shift-right: [w287] -> _
    shift-left: _ -> [w288]
    tunnel: w4 -> [w285]
    tunnel: w3 -> [w284]
    tunnel: w2 -> [w282]
    tunnel: "TopLevel" -> [w280]
    stop <- w292 stop-if-true
    n104 = call <vilib>:"Parse State Queue__JKI_lib_State_Machine.vi"("State Queue"=w295, "Error In (no error)"=w289) -> ("Remaining States"=w297:string, "Current State"=w283:string, "Arguments"=w296:string)  [unwired: 11 in]
    n105 = feedback #1(w282) -> (w281:string)
    n106 = feedback-in #1(w283) -> ()
    n107 = case shown="\"Process Sync\"" w283 {
      selector: w283 -> [w298 _ _ _ _ _ _ _ _ _ _ _ _ _ _ _ _ _ _ _ _ _ _ _ _ _ _]
      tunnel: w297 -> [w305 w315 w417 w434 w443 w458 w464 w480 w516 w519 w526 w534 w537 w550 w555 w558 w581 w616 w650 w684 w697 w704 w715 w734 w765 w780 w793]
      tunnel: w296 -> [_ _ _ _ _ _ _ _ _ _ _ _ _ _ _ _ _ _ _ _ _ _ _ w730 _ _ _]
      tunnel: w290 -> [w306 w313 w415 w429 w444 w453 w463 w476 w505 w518 w523 w530 w536 w548 w554 w557 w571 w613 w647 w681 w696 w699 w712 w724 w763 w774 w792]
      tunnel: [w299 w312 w406 w428 w445 w460 w465 w477 w501 w520 w524 w532 w538 w547 w551 w559 w563 w607 w641 w675 w698 w700 w710 w726 w761 w776 w794] -> w294
      tunnel: w289 -> [_ w311 w413 w431 w446 w460 w465 w469 w507 w520 w524 w532 w538 w539 w551 w559 w564 w608 w642 w676 w698 w701 w711 w727 w762 w768 w794]
      tunnel: [w305 w314 w417 w433 w443 w458 w464 w480 w516 w519 w525 w533 w537 w550 w555 w558 w581 w616 w650 w684 w697 w704 w715 w734 w765 w780 w793] -> w293
      tunnel: [_ _ _ _ _ TRUE _ _ _ _ _ _ _ _ _ _ _ _ _ _ _ _ _ _ _ _ _] -> w292
      tunnel: [w306 w310 w415 w429 w444 w453 w463 w476 w512 w518 w523 w529 w536 w548 w554 w557 w571 w613 w647 w681 w696 w699 w712 w724 w763 w774 w792] -> w291
      tunnel: w288 -> [w304 w309 w416 w432 w442 w457 w462 w479 w515 w517 w522 w531 w535 _ w552 w556 w580 w615 w649 w683 w695 w703 w714 w733 w764 w779 w791]
      tunnel: [w304 w308 w416 w432 w442 w457 w462 w479 w515 w517 w522 w531 w535 w549 w552 w556 w580 w615 w649 w683 w695 w703 w714 w733 w764 w779 w791] -> w287
      tunnel: 100 ("Timeout") -> [_ w307 _ _ _ _ _ _ _ _ _ _ _ _ _ _ _ _ _ _ _ _ _ _ _ _ _]
      tunnel: w281 -> [_ _ _ w430 _ _ _ _ _ _ _ _ _ _ _ _ _ _ _ _ _ _ _ _ _ _ _]
      tunnel: w285 -> [_ _ _ _ _ _ _ _ _ _ w521 _ _ _ _ _ _ _ _ _ _ _ _ _ _ _ _]
      tunnel: w284 -> [_ _ _ _ _ _ _ _ _ _ _ w527 _ _ _ _ _ _ _ _ _ _ _ _ _ _ _]
      tunnel: w280 -> [_ _ w404 _ _ _ _ _ _ _ _ _ _ w543 _ _ _ _ _ _ _ _ _ _ _ _ _]
      frame Default {
        # "Do not delete, rename, or modify this frame. (this is used to capture unhandled states and typos)"
        n108 = Format Into String(format string="Software Exception: \nUnhandled State: \"%s\"", w298) -> (resulting string=w302:string)  [unwired: 2 in, 1 out]
        n109 = call <vilib>:"Build Error Cluster_ModKT .vi"("Prepend String (\"\")"=w302, "code"=5001, "error? (F)"=TRUE ("error?")) -> ("error out"=w299:errorcluster)  [unwired: 4 in, 1 out]
      }
      frame "", "Event Handler", "Idle" {
        n110 = event "executes when the state queue is empty" shown="[1] <Exit Event>: User Event" {
          selector: w309 -> [_ _ _ _ _ _ _ _]
          dyn-events: [_ _ _ _ _ _ _ _] -> w308
          timeout: w307 -> [_ _ _ _ _ _ _ _]
          tunnel: w315 -> [w317 w328 _ w337 w350 w368 w399 w402]
          tunnel: [w316 w329 w333 w339 w349 w367 w399 w402] -> w314
          tunnel: w313 -> [w318 w330 w335 w340 w348 w365 w398 w401]
          tunnel: [w319 w331 w336 w341 w358 w369 w397 "injected error cluster"] -> w312
          tunnel: w311 -> [w319 w331 w336 w341 w358 w370 w397 _]
          tunnel: [w318 w330 w334 w340 w347 w364 w398 w401] -> w310
          event Timeout {
            n111 = event-data() -> ()  [unwired: 1 in, 1 out]
            n112 = disable-structure shown="Enabled" {
              disable-tunnel: w317 -> [w321 w326]
              disable-tunnel: [w320 w326] -> w316
              frame Disabled {
                n113 = disable-structure shown="Disabled" {
                  disable-tunnel: ["Loop: Read Data" _] -> w322
                  frame Disabled {
                  }
                  frame Enabled {
                  }
                }
                n114 = call <userlib>:"Periodic Trigger__ogtk.vi"("time (ms)"=u32 1000) -> ("Triggered"=w323:bool)  [unwired: 12 in, 2 out]
                n115 = Select(t=w322, s=w323, f=w321) -> (s? t:f=w320:string)
              }
              frame Enabled {
              }
            }
          }
          event User Event {
            n116 = event-data() -> ()  [unwired: 1 in, 5 out]
            n117 = call <vilib>:"Add State(s) to Queue__JKI_lib_State_Machine.vi"("State(s) in Front (\"\")"="Macro: Exit" ("State(s) in Front (\"\")"), "State(s) in (\"\")"=w328) -> ("States Out"=w329:string)  [unwired: 13 in]
          }
          event User Event {
            w333 = "Macro: Exit"  # Macro: Exit
            # "This notifier needs to be fired as the last step of the exit macro sequence. This is the handshaking."
            n118 = event-data() -> ("notifier out"=w332:refnum<notifier>)  [unwired: 1 in]
            n119 = Bundle By Name(cluster=w335, "Core.process sync notifier"=w332) -> (w334:T1)
          }
          event "Stop Process": Value Change {
            n120 = event-data() -> ()  [unwired: 1 in, 1 out]
            n121 = call <vilib>:"Add State(s) to Queue__JKI_lib_State_Machine.vi"("State(s) in Front (\"\")"="Macro: Exit", "State(s) in (\"\")"=w337) -> ("States Out"=w339:string)  [unwired: 13 in]
          }
          event User Event {
            w357 = T10 {"TimeStamp"=0.0, "DaqOutCmd"=enum."Set DO", "IOName"="", "BoolState"=FALSE, "AnalogVal"=0.0, "WaitTime (ms)"=0, "mode"=enum."manual", "vData"=variant}  # DaqOutputCmd
            n122 = event-data() -> ("TimeStamp"=w356:dbl, "DaqOutCmd"=w345:T11, "IOName"=w355:string, "BoolState"=w354:bool, "AnalogVal"=w353:dbl, "WaitTime (ms)"=w352:u32, "mode"=w343:T12, "vData"=w342:variant)  [unwired: 1 in]
            n123 = Bundle By Name(cluster=w357, "TimeStamp"=w356, "DaqOutCmd"=w345, "IOName"=w355, "BoolState"=w354, "AnalogVal"=w353, "WaitTime (ms)"=w352, "mode"=w343, "vData"=w342) -> (w351:T10)
            n124 = case shown="\"Invert DO\"" w345 {
              tunnel: ["Prep: Set DO" "Prep: Set AO" "Prep: Toggle DO" "Prep: Invert DO"] -> w344
              frame "Set DO", Default {
              }
              frame "Set AO" {
              }
              frame "Toggle DO" {
              }
              frame "Invert DO" {
              }
            }
            n125 = To Variant(anything=w351) -> (Variant=w346:variant)
            n126 = Bundle By Name(cluster=w348, "vData"=w346) -> (w347:T1)
            n127 = call <vilib>:"Add State(s) to Queue__JKI_lib_State_Machine.vi"("State(s) in Front (\"\")"=w344, "State(s) in (\"\")"=w350) -> ("States Out"=w349:string)  [unwired: 13 in]
          }
          event User Event {
            w363 = AsyncCmd_DAQ--enum."StartDAQ" ("AsyncMsg")
            n128 = event-data() -> ("CmdMsg"=w371:string, "vData"=w372:variant)  [unwired: 1 in, 1 out]
            n129 = call <userlib>:"Set Enum String Value__ogtk.vi"("error in (no error)"=w370, "String Value"=w371, "Default Enum Value"=w363) -> ("error out"=w374:errorcluster, "Enum"=w373:variant)  [unwired: 7 in]
            n130 = Variant To Data(error in=w374, type=w363, Variant=w373) -> (data=w375:T15, error out=w376:errorcluster)
            n131 = case shown="Default" w375 {
              selector: w375 -> [_ w391 _]
              tunnel: w372 -> [_ w384 w394]
              tunnel: w376 -> [w381 w387 w393]
              tunnel: [w380 w388 w393] -> w369
              tunnel: ["" w389 "Action: CfgDAQ\nIdle"] -> w366
              tunnel: w365 -> [w383 w385 w395]
              tunnel: [w383 w386 w396] -> w364
              frame Default {
                n132 = call <vilib>:"Build Error Cluster_ModKT .vi"("Prepend String (\"\")"="Bad Cmd" ("Prepend String (\"\")"), "code"=42, "error? (F)"=TRUE, "error in (no error)"=w381) -> ("error out"=w380:errorcluster)  [unwired: 3 in, 1 out]
              }
              frame "StartDAQ", "StopDAQ" {
                # "NOTE: Start or Stop all AI DAQ SM's"
                n133 = Format Into String(format string="Action: StartStopDAQ >> %s\nIdle", error in=w387, w391) -> (resulting string=w389:string, error out=w388:errorcluster)  [unwired: 1 in]
                n134 = Bundle By Name(cluster=w385, "vData"=w384) -> (w386:T1)
              }
              frame "CfgDAQ" {
                # "#TODO:  finish implementing\nCfgDaq params to reconfigure\nDAQ settings (sample rate / num samples)"
                n135 = Bundle By Name(cluster=w395, "vData"=w394) -> (w396:T1)
              }
            }
            n136 = call <vilib>:"Add State(s) to Queue__JKI_lib_State_Machine.vi"("State(s) in Front (\"\")"=w366, "State(s) in (\"\")"=w368) -> ("States Out"=w367:string)  [unwired: 13 in]
          }
          event User Event {
            n137 = event-data() -> ()  [unwired: 1 in, 3 out]
          }
          event "inject error": Value Change {
            n138 = event-data() -> ()  [unwired: 1 in, 6 out]
          }
        }
      }
      frame "Process Sync" {
        # "#TODO AD fix this after deleting"
        # "KT 2018-0211\nuncommented DAQ thread's ThreadSync at shutdown"
        # "Rendezvous sync with DAQ\nthreads; only for startup,\nnot shutdown"
        n139 = Unbundle By Name(w415) -> ("Core.process sync notifier"=w414:refnum<notifier>, "ThreadSyncRndzv"=w410:T7)  [unwired: 1 out]
        n140 = property class="TopLevel.lvclass"(reference=w404) -> ("Methods:Accessors:StatusStrRef"=w403:refnum<vi>)  [unwired: 1 in, 2 out]
        n141 = case shown="False" FALSE {
          tunnel: w413 -> [w425 w427]
          tunnel: [w424 w427] -> w412
          tunnel: w410 -> [w423 _]
          frame False {
            # "timeout up to 1 min"
            n142 = call <vilib>:"Wait at Rendezvous.vi"("error in (no error)"=w425, "ms timeout (-1)"=60000, "rendezvous"=w423) -> ("error out"=w424:errorcluster)  [unwired: 2 in, 2 out]
          }
          frame True {
          }
        }
        n143 = call <vilib>:"format status message v2.vi"("status msg"="Launched DAQ Module", "Str Refnum"=w403) -> ()  [unwired: 5 in, 5 out]
        n144 = call <userlib>:"Wait (ms)__ogtk.vi"("error in (no error)"=w412, "milliseconds to wait"=u32 2000) -> ("error out"=w408:errorcluster)  [unwired: 8 in, 1 out]
        n145 = disable-structure shown="Enabled" {
          disable-tunnel: w414 -> [w421 _]
          disable-tunnel: [w420 w422] -> w411
          disable-tunnel: w408 -> [w418 w422]
          frame Enabled {
            n146 = Send Notification(notification=TRUE, notifier=w421, error in (no error)=w418) -> (error out=w420:errorcluster)  [unwired: 1 out]
          }
          frame Disabled {
          }
        }
        n147 = call <vilib>:"Clear Errors.vi"("error in (no error)"=w411) -> ("error out"=w406:errorcluster)  [unwired: 5 in, 1 out]
      }
      frame "Error Handler" {
        n148 = disable-structure shown="Enabled" {
          disable-tunnel: w431 -> [w439 w441]
          disable-tunnel: w430 -> [w438 _]
          disable-tunnel: [w437 errorcluster {"status"=FALSE, "code"=0, "source"=""} ("error constant")] -> w428
          frame Enabled {
            n149 = Concatenate Strings("Previous State: ", w438) -> (w435:string)
            n150 = call "Handle Error SM.vi"("error in (no error)"=w439, "CustomMessage"=w435) -> ("error out"=w437:errorcluster)  [unwired: 7 in, 2 out]
          }
          frame Disabled {
            n151 = call <vilib>:"General Error Handler.vi"("error in (no error)"=w441) -> ()  [unwired: 10 in, 5 out]
          }
        }
        n152 = call <vilib>:"Add State(s) to Queue__JKI_lib_State_Machine.vi"("State(s) in (\"\")"=w434) -> ("States Out"=w433:string)  [unwired: 14 in]
      }
      frame "CleanUp" {
        # "Cleanup any data and references, here. (this is called automatically, by the Macro: Exit)"
        n153 = Unbundle By Name(w444) -> ("Core.Current VI Ref"=w447:refnum<vi>)
        n154 = Close Reference(reference=w447, error in (no error)=w446) -> (error out=w445:errorcluster)
      }
      frame "Exit", "Quit" {
        n155 = Unbundle By Name(w453) -> ("ThreadSyncRndzv"=w451:T7, "AI Thread SMQs"=w454:variant, "DI Thread SMQs"=w449:variant)
        n156 = Delete Variant Attribute(7:w454) -> (0:w455:errorcluster, 3:w456:variant)  [unwired: 2 in, 1 out]
        n157 = Delete Variant Attribute(7:w449) -> (0:w450:errorcluster)  [unwired: 2 in, 2 out]
        n158 = call <userlib>:"Clear All Errors__ogtk.vi"("Error In"=w455) -> ("Error Out"=w452:errorcluster)  [unwired: 3 in]
        n159 = call <userlib>:"Clear All Errors__ogtk.vi"("Error In"=w450) -> ("Error Out"=w448:errorcluster)  [unwired: 3 in]
        n160 = flat-sequence {
          tunnel: w456 -> [_]
          tunnel: w452 -> [_]
          tunnel: w451 -> [w461]
          tunnel: w448 -> [_]
          frame #0 {
            n161 = call <vilib>:"Destroy Rendezvous.vi"("rendezvous"=w461) -> ()  [unwired: 5 in, 2 out]
          }
        }
      }
      frame "------ Data ------" {
      }
      frame "Data: SetDaqOutValues" {
        n162 = Unbundle By Name(w476) -> ("Self Reference"=w475:refnum<class "DAQ.lvclass">)
        n163 = property class="DAQ"(reference=w475, error in=w469) -> (reference out=w470:refnum<class "DAQ.lvclass">, error out=w468:errorcluster, "Accessors:IO Nodes"=w472:T16)
        n164 = Unbundle By Name(w472) -> ("AO Config.AO Channels"=w473:T13[], "DO Config.DO Channels"=w474:T9[])
        n165 = for {
          tunnel: w473 -> [w484] mode=indexing
          tunnel: [w483] -> w466 mode=indexing
          n166 = Unbundle By Name(w484) -> ("IOName"=w483:string)
        }
        n167 = for {
          tunnel: w474 -> [w482] mode=indexing
          tunnel: [w481] -> w467 mode=indexing
          n168 = Unbundle By Name(w482) -> ("IOName"=w481:string)
        }
        n169 = for {
          tunnel: w467 -> [w494] mode=indexing
          shift-right: [w497] -> w471
          shift-left: w468 -> [w496]
          shift-right: [w492] -> w478
          shift-left: w470 -> [w493]
          n170 = call "Read DO Data Value.vi"("error in (no error)"=w496, "Name"=w494, "DAQ"=w493) -> ("error out"=w498:errorcluster, "state"=w495:bool, "DAQ"=w499:refnum<class "DAQ.lvclass">)  [unwired: 6 in]
          n171 = call "Set DAQ Boolean Data Value.vi"("DAQ"=w499, "Value"=w495, "Name"=w494, "error in (no error)"=w498) -> ("DAQ"=w492:refnum<class "DAQ.lvclass">, "error out"=w497:errorcluster)  [unwired: 9 in, 1 out]
        }
        n172 = for {
          tunnel: w466 -> [w487] mode=indexing
          shift-right: [w489] -> w477
          shift-left: w471 -> [w488]
          tunnel: w478 -> [w486]
          n173 = call "Read AO Data Value.vi"("error in (no error)"=w488, "Name"=w487, "DAQ"=w486) -> ("error out"=w490:errorcluster, "data value"=w485:dbl, "DAQ"=w491:refnum<class "DAQ.lvclass">)  [unwired: 6 in]
          n174 = call "Set DAQ Analog Data Value.vi"("DAQ"=w491, "Value"=w485, "Name"=w487, "error in (no error)"=w490) -> ("error out"=w489:errorcluster)  [unwired: 9 in, 2 out]
        }
      }
      frame "Data: Initialize" {
        n175 = Unbundle By Name(w505) -> ("AI Thread SMQs"=w510:variant, "Self Reference"=w508:refnum<class "DAQ.lvclass">)
        n176 = Unbundle By Name(w505) -> ("DI Thread SMQs"=w504:variant)
        n177 = property class="DAQ"(reference=w508) -> ("Accessors:AI TaskNames*"=w509:string[], "Accessors:DI TaskNames*"=w503:string[])  [unwired: 1 in, 2 out]
        n178 = call-poly "Get AI DAQ SMQ - polymorphic.vi"("error in (no error)"=w507, "AI TaskNames"=w509, "AI Thread SMQs"=w510) -> ("error out"=w502:errorcluster, "AI DAQ SMQ []"=w506:refnum<queue>[])  [unwired: 6 in, 1 out]
        n179 = call-poly "Get DI DAQ SMQ - polymorphic.vi"("error in (no error)"=w502, "AI TaskNames"=w503, "AI Thread SMQs"=w504) -> ("error out"=w501:errorcluster, "AI DAQ SMQ []"=w500:refnum<queue>[])  [unwired: 6 in, 1 out]
        n180 = control-ref of="Current VI Reference"() -> (w514:refnum<vi>)
        n181 = Bundle By Name(cluster=w505, "Core.Current VI Ref"=w514, "Core.process sync notifier"="start process sync notifier", "quitting"=FALSE, "AI DAQ SMQ []"=w506, "DI DAQ SMQ []"=w500) -> (w512:T1)
      }
      frame "------ Macro ------" {
      }
      frame "Macro: Initialize" {
        # "Initialization Macro (This is called once, when the VI starts)"
        n182 = call <vilib>:"Add State(s) to Queue__JKI_lib_State_Machine.vi"("State(s) in Front (\"\")"=w521, "State(s) in (\"\")"=w526) -> ("States Out"=w525:string)  [unwired: 13 in]
      }
      frame "Macro: Exit" {
        n183 = Bundle By Name(cluster=w530, "quitting"=TRUE) -> (w529:T1)
        n184 = call <vilib>:"Add State(s) to Queue__JKI_lib_State_Machine.vi"("State(s) in Front (\"\")"=w527, "State(s) in (\"\")"=w534) -> ("States Out"=w533:string)  [unwired: 13 in]
      }
      frame "------ UI ------" {
      }
      frame "UI: Register Events" {
        n185 = Unbundle By Name(w548) -> ("Self Reference"=w545:refnum<class "DAQ.lvclass">)
        n186 = call-dynamic "GetEvents_TopLevel.vi"("error in (no error)"=w539, "TopLevel in"=w543) -> ("error out"=w540:errorcluster, "UserEvents"=w542:T27)  [unwired: 7 in, 1 out]
        n187 = call "Get Public Events.vi"("error in (no error)"=w540, "DAQ"=w545) -> ("error out"=w544:errorcluster, "PublicEvents"=w546:T28)  [unwired: 7 in, 1 out]
        n188 = Unbundle By Name(w542) -> ("Exit Event"=w541:refnum<user-event>)
        n189 = register-events(error in=w544, w546, w541) -> (reference out=w549:refnum<event-registration>, error out=w547:errorcluster)  [unwired: 1 in]
      }
      frame "UI: Unregister Events" {
        n190 = Unregister For Events(event registration refnum=w552, error in=w551) -> (error out=w553:errorcluster)
        n191 = call <vilib>:"Clear Errors.vi"("error in (no error)"=w553) -> ()  [unwired: 5 in, 2 out]
      }
      frame "------ Prep ------" {
      }
      frame "Prep: Set AO" {
        w569 = T10 {"TimeStamp"=0.0, "DaqOutCmd"=enum."Set DO", "IOName"="", "BoolState"=FALSE, "AnalogVal"=0.0, "WaitTime (ms)"=0, "mode"=enum."manual", "vData"=variant}  # DaqOutputCmd
        # "used for updating\nmain status string\nif applicable"
        n192 = Unbundle By Name(w571) -> ("AsyncSMQ"=w566:refnum<queue>, "DAQ Node Dict DVR"=w568:T8)
        n193 = Unbundle By Name(w571) -> ("vData"=w570:variant)
        n194 = Variant To Data(error in=w564, type=w569, Variant=w570) -> (data=w561:T10, error out=w572:errorcluster)
        n195 = Unbundle By Name(w561) -> ("mode"=w560:T12)
        n196 = in-place {
          in-place-border: w572 -> [w587]
          in-place-border: [w586] -> w574
          in-place-border: w568 -> [w591]
          in-place-border: [w584] -> w575
          in-place-border: [w588] -> w573
          in-place-border: [w590] -> _
          in-place-border: w561 -> [w592]
          in-place-border: [w592] -> w579
          n197 = in-place-cluster #2(w561) -> ("IOName"=w589:string, "AnalogVal"=w588:dbl)
          n198 = call "Retrieve Scaling and Convert AO to RawVal.vi"("error in (no error)"=w587, "EU Value in"=w588, "IOName"=w589, "DaqDevice dCVT"=w591) -> ("error out"=w586:errorcluster, "Raw Value Out"=w585:dbl, "IOName out"=w584:string, "In Range?"=w590:bool)  [unwired: 3 in, 1 out]
          n199 = in-place-cluster #2("IOName"=w584, "AnalogVal"=w585) -> (w577:T10)
        }
        n200 = Bundle("DaqOutputCmd"=w579, "DaqOutputCmd"=w577) -> (w578:cluster{"DaqOutputCmd":T10, "DaqOutputCmd":T10})  [unwired: 1 in]
        n201 = Format Into String(format string=" : %f", initial string=w575, error in=w574, w573) -> (error out=w565:errorcluster)  [unwired: 1 out]
        n202 = To Variant(anything=w578) -> (Variant=w567:variant)
        n203 = case shown="\"automation\"" w560 {
          tunnel: ["Cmd: Set AO" "Cmd: Set AO >> UpdCtrl"] -> w562
          frame "manual", Default {
          }
          frame "automation" {
          }
        }
        n204 = call <vilib>:"Add State to Queue with vData.vi"("queue in"=w566, "state in"=w562, "vData (\"\")"=w567, "error in"=w565) -> ("error out"=w563:errorcluster)  [unwired: 8 in, 3 out]
      }
      frame "Prep: Set DO" {
        w611 = T10 {"TimeStamp"=0.0, "DaqOutCmd"=enum."Set DO", "IOName"="", "BoolState"=FALSE, "AnalogVal"=0.0, "WaitTime (ms)"=0, "mode"=enum."manual", "vData"=variant}  # DaqOutputCmd
        # "used for updating\nmain status string\nif applicable"
        n205 = Unbundle By Name(w613) -> ("AsyncSMQ"=w609:refnum<queue>, "DAQ Node Dict DVR"=w606:T8)
        n206 = Unbundle By Name(w613) -> ("vData"=w612:variant)
        n207 = Variant To Data(error in=w608, type=w611, Variant=w612) -> (data=w595:T10, error out=w603:errorcluster)
        n208 = Unbundle By Name(w595) -> ("mode"=w594:T12)
        n209 = in-place {
          in-place-border: w603 -> [w626]
          in-place-border: [w625] -> w602
          in-place-border: w606 -> [w624]
          in-place-border: [w622] -> w597
          in-place-border: [w620] -> w596
          in-place-border: w595 -> [w619]
          in-place-border: [w619] -> w605
          n210 = in-place-cluster #3(w595) -> ("IOName"=w623:string, "BoolState"=w620:bool)
          n211 = call "Retrieve Logic and Convert DO.vi"("error in (no error)"=w626, "StateValue in"=w620, "IOName"=w623, "DAQ Node Dict DVR"=w624) -> ("error out"=w625:errorcluster, "ConvertedValue Out"=w621:bool, "IOName out"=w622:string)  [unwired: 4 in, 1 out]
          n212 = in-place-cluster #3("IOName"=w622, "BoolState"=w621) -> (w604:T10)
        }
        n213 = Bundle("DaqOutputCmd"=w605, "DaqOutputCmd"=w604) -> (w614:cluster{"DaqOutputCmd":T10, "DaqOutputCmd":T10})  [unwired: 1 in]
        n214 = To Variant(anything=w614) -> (Variant=w610:variant)
        n215 = Select(t=" : Close", s=w596, f=": Open") -> (s? t:f=w600:string)
        n216 = case shown="\"manual\", Default" w594 {
          tunnel: ["Cmd: Set DO" "Cmd: Set DO >> UpdCtrl"] -> w593
          frame "manual", Default {
          }
          frame "automation" {
          }
        }
        n217 = Concatenate Strings("\r\n", w597, w600) -> ()  [unwired: 1 out]
        n218 = call <vilib>:"Add State to Queue with vData.vi"("queue in"=w609, "state in"=w593, "vData (\"\")"=w610, "error in"=w602) -> ("error out"=w607:errorcluster)  [unwired: 8 in, 3 out]
      }
      frame "Prep: Toggle DO" {
        w645 = T10 {"TimeStamp"=0.0, "DaqOutCmd"=enum."Set DO", "IOName"="", "BoolState"=FALSE, "AnalogVal"=0.0, "WaitTime (ms)"=0, "mode"=enum."manual", "vData"=variant}  # DaqOutputCmd
        # "used for updating\nmain status string\nif applicable"
        n219 = Unbundle By Name(w647) -> ("AsyncSMQ"=w643:refnum<queue>, "DAQ Node Dict DVR"=w640:T8)
        n220 = Unbundle By Name(w647) -> ("vData"=w646:variant)
        n221 = Variant To Data(error in=w642, type=w645, Variant=w646) -> (data=w629:T10, error out=w637:errorcluster)
        n222 = Unbundle By Name(w629) -> ("mode"=w628:T12)
        n223 = in-place {
          in-place-border: w637 -> [w660]
          in-place-border: [w659] -> w636
          in-place-border: w640 -> [w658]
          in-place-border: [w656] -> w631
          in-place-border: [w654] -> w630
          in-place-border: w629 -> [w653]
          in-place-border: [w653] -> w639
          n224 = in-place-cluster #4(w629) -> ("IOName"=w657:string, "BoolState"=w654:bool)
          n225 = call "Retrieve Logic and Convert DO.vi"("error in (no error)"=w660, "StateValue in"=w654, "IOName"=w657, "DAQ Node Dict DVR"=w658) -> ("error out"=w659:errorcluster, "ConvertedValue Out"=w655:bool, "IOName out"=w656:string)  [unwired: 4 in, 1 out]
          n226 = in-place-cluster #4("IOName"=w656, "BoolState"=w655) -> (w638:T10)
        }
        n227 = Bundle("DaqOutputCmd"=w639, "DaqOutputCmd"=w638) -> (w648:cluster{"DaqOutputCmd":T10, "DaqOutputCmd":T10})  [unwired: 1 in]
        n228 = case shown="\"automation\"" w628 {
          tunnel: ["Cmd: Toggle DO" "Cmd: Toggle DO >> UpdCtrl"] -> w627
          frame "manual", Default {
          }
          frame "automation" {
          }
        }
        n229 = To Variant(anything=w648) -> (Variant=w644:variant)
        n230 = Select(t=" : Close", s=w630, f=": Open") -> (s? t:f=w634:string)
        n231 = Concatenate Strings("\r\n", w631, w634) -> ()  [unwired: 1 out]
        n232 = call <vilib>:"Add State to Queue with vData.vi"("queue in"=w643, "state in"=w627, "vData (\"\")"=w644, "error in"=w636) -> ("error out"=w641:errorcluster)  [unwired: 8 in, 3 out]
      }
      frame "Prep: Invert DO" {
        w679 = T10 {"TimeStamp"=0.0, "DaqOutCmd"=enum."Set DO", "IOName"="", "BoolState"=FALSE, "AnalogVal"=0.0, "WaitTime (ms)"=0, "mode"=enum."manual", "vData"=variant}  # DaqOutputCmd
        # "used for updating\nmain status string\nif applicable"
        n233 = Unbundle By Name(w681) -> ("AsyncSMQ"=w677:refnum<queue>, "DAQ Node Dict DVR"=w674:T8)
        n234 = Unbundle By Name(w681) -> ("vData"=w680:variant)
        n235 = Variant To Data(error in=w676, type=w679, Variant=w680) -> (data=w663:T10, error out=w671:errorcluster)
        n236 = Unbundle By Name(w663) -> ("mode"=w662:T12)
        n237 = in-place {
          in-place-border: w671 -> [w694]
          in-place-border: [w693] -> w670
          in-place-border: w674 -> [w692]
          in-place-border: [w690] -> w665
          in-place-border: [w688] -> w664
          in-place-border: w663 -> [w687]
          in-place-border: [w687] -> w673
          n238 = in-place-cluster #5(w663) -> ("IOName"=w691:string, "BoolState"=w688:bool)
          n239 = call "Retrieve Logic and Convert DO.vi"("error in (no error)"=w694, "StateValue in"=w688, "IOName"=w691, "DAQ Node Dict DVR"=w692) -> ("error out"=w693:errorcluster, "ConvertedValue Out"=w689:bool, "IOName out"=w690:string)  [unwired: 4 in, 1 out]
          n240 = in-place-cluster #5("IOName"=w690, "BoolState"=w689) -> (w672:T10)
        }
        n241 = Bundle("DaqOutputCmd"=w673, "DaqOutputCmd"=w672) -> (w682:cluster{"DaqOutputCmd":T10, "DaqOutputCmd":T10})  [unwired: 1 in]
        n242 = case shown="\"automation\"" w662 {
          tunnel: ["Cmd: Invert DO" "Cmd: Invert DO >> UpdCtrl"] -> w661
          frame "manual", Default {
          }
          frame "automation" {
          }
        }
        n243 = To Variant(anything=w682) -> (Variant=w678:variant)
        n244 = Select(t=" : Close", s=w664, f=": Open") -> (s? t:f=w668:string)
        n245 = Concatenate Strings("\r\n", w665, w668) -> ()  [unwired: 1 out]
        n246 = call <vilib>:"Add State to Queue with vData.vi"("queue in"=w677, "state in"=w661, "vData (\"\")"=w678, "error in"=w670) -> ("error out"=w675:errorcluster)  [unwired: 8 in, 3 out]
      }
      frame "------ Action ------" {
      }
      frame "Action: Launch SM AI Threads" {
        # "#AItasks"
        n247 = Unbundle By Name(w699) -> ("Self Reference"=w702:refnum<class "DAQ.lvclass">)
        n248 = disable-structure shown="Enabled" {
          disable-tunnel: w702 -> [w708 _]
          disable-tunnel: w701 -> [w707 w709]
          disable-tunnel: [w706 w709] -> w700
          disable-tunnel: w699 -> [w705 _]
          frame Enabled {
            n249 = call "Launch SM AI Threads.vi"("error in (no error)"=w707, "DAQ Process AppData"=w705, "DAQ in"=w708) -> ("error out"=w706:errorcluster)  [unwired: 7 in, 1 out]
          }
          frame Disabled {
          }
        }
      }
      frame "Action: Launch SM DI Threads" {
        # "#DItasks"
        n250 = Unbundle By Name(w712) -> ("Self Reference"=w713:refnum<class "DAQ.lvclass">)
        n251 = disable-structure shown="Enabled" {
          disable-tunnel: w713 -> [w719 _]
          disable-tunnel: w712 -> [w718 _]
          disable-tunnel: w711 -> [w717 w720]
          disable-tunnel: [w716 w720] -> w710
          frame Enabled {
            n252 = call "Launch SM DI Threads.vi"("error in (no error)"=w717, "DAQ Process AppData"=w718, "DAQ in"=w719) -> ("error out"=w716:errorcluster)  [unwired: 7 in, 1 out]
          }
          frame Disabled {
          }
        }
      }
      frame "Action: StartStopDAQ" {
        # "NOTE: Start or Stop all AI & DI DAQ SM's"
        n253 = Unbundle By Name(w724) -> ("DI DAQ SMQ []"=w723:refnum<queue>[], "vData"=w722:variant)
        n254 = Format Into String(format string="Macro: %s", w730) -> (resulting string=w721:string)  [unwired: 2 in, 1 out]
        n255 = disable-structure shown="Disabled" {
          disable-tunnel: w724 -> [w745 _]
          frame Disabled {
            n256 = Unbundle By Name(w745) -> ("DAQ Settings.AI Settings"=w744:T4[])
            n257 = Index Array(array=w744) -> (element=w743:T4)  [unwired: 1 in]
            n258 = Unbundle By Name(w743) -> ("AI InstSettings.DaqRate"=w741:dbl, "AI InstSettings.NumSamples"=w742:i32)
            n259 = Divide(x=w742, y=w741) -> (x/y=→"time per buffer":dbl)
          }
          frame Enabled {
          }
        }
        n260 = Unbundle By Name(w724) -> ("AI DAQ SMQ []"=w732:refnum<queue>[], "vData"=w728:variant)
        n261 = for {
          tunnel: w732 -> [w750] mode=indexing
          tunnel: w721 -> [w749]
          tunnel: w728 -> [w748]
          shift-right: [w747] -> w731
          shift-left: w727 -> [w746]
          n262 = call <vilib>:"Add State to Queue with vData.vi"("queue in"=w750, "state in"=w749, "vData (\"\")"=w748, "error in"=w746) -> ("error out"=w747:errorcluster)  [unwired: 8 in, 3 out]
        }
        n263 = for {
          tunnel: w723 -> [w739] mode=indexing
          tunnel: w721 -> [w738]
          tunnel: w722 -> [w737]
          shift-right: [w736] -> w725
          shift-left: w727 -> [w735]
          n264 = call <vilib>:"Add State to Queue with vData.vi"("queue in"=w739, "state in"=w738, "vData (\"\")"=w737, "error in"=w735) -> ("error out"=w736:errorcluster)  [unwired: 8 in, 3 out]
        }
        n265 = Merge Errors(w731, w725) -> (w726:errorcluster)
      }
      frame "Action: CfgDAQ" {
        # "#TODO:  finish implementing\nCfgDaq params to reconfigure\nDAQ settings (sample rate / num samples)"
        n266 = Unbundle By Name(w763) -> ("AI Thread SMQs"=w758:variant, "vData"=w759:variant)
        n267 = Bundle("AI InstSettings"=T5 {"DaqRate"=0.0, "NumSamples"=0}, "AI TaskName"="") -> (w755:T29)  [unwired: 1 in]
        n268 = Variant To Data(type=w755, Variant=w759) -> (data=w754:T29)  [unwired: 1 in, 1 out]
        n269 = Unbundle(w754) -> ("AI InstSettings"=w753:T5, "AI TaskName"=w752:string)
        n270 = call-poly "Get AI DAQ SMQ - polymorphic.vi"("AI TaskName"=w752, "AI Thread SMQs"=w758) -> ("AI DAQ SMQ"=w751:refnum<queue>)  [unwired: 7 in, 2 out]
        n271 = call <vilib>:"Add State to Queue with vData.vi"("queue in"=w751, "state in"="Macro: CfgDAQ", "vData (\"\")"=w753, "error in"=w762) -> ("error out"=w761:errorcluster)  [unwired: 8 in, 3 out]
      }
      frame "Action: TerminateAsyncThreads" {
        w769 = enum16{"back", "front"}."front" ("mode (back)")
        n272 = Unbundle By Name(w774) -> ("AsyncSMQ"=w778:refnum<queue>, "DI DAQ SMQ []"=w770:refnum<queue>[], "AI DAQ SMQ []"=w772:refnum<queue>[])
        n273 = for {
          tunnel: w769 -> [w788]
          shift-right: [w787] -> w766
          shift-left: w768 -> [w790]
          tunnel: w772 -> [w786] mode=indexing
          n274 = call <vilib>:"Add State to Queue with vData.vi"("queue in"=w786, "mode (back)"=w788, "state in"="Macro: Exit", "error in"=w790) -> ("error out"=w787:errorcluster)  [unwired: 8 in, 3 out]
        }
        n275 = for {
          tunnel: w769 -> [w783]
          shift-right: [w782] -> w771
          shift-left: w768 -> [w785]
          tunnel: w770 -> [w781] mode=indexing
          n276 = call <vilib>:"Add State to Queue with vData.vi"("queue in"=w781, "mode (back)"=w783, "state in"="Macro: Exit", "error in"=w785) -> ("error out"=w782:errorcluster)  [unwired: 8 in, 3 out]
        }
        n277 = Merge Errors(w771, w766) -> (w767:errorcluster)
        n278 = call <vilib>:"Add State to Queue with vData.vi"("queue in"=w778, "mode (back)"=w769, "state in"="CleanUp", "error in"=w767) -> ("error out"=w777:errorcluster)  [unwired: 8 in, 3 out]
        n279 = call <userlib>:"Wait (ms)__ogtk.vi"("error in (no error)"=w777, "milliseconds to wait"=u32 1000) -> ("error out"=w776:errorcluster)  [unwired: 8 in, 1 out]
      }
      frame "Loop: Read Data" {
      }
    }
  }
  n280 = Merge Errors(w6, w7) -> (→"error out":errorcluster)
